vi "Enclose with Diagram Disable Structure Target.vi"(11 "Input":bool[](array[boolean])) -> (3 "Any?":bool)   [LabVIEW 2018, in "Tests.lvlib" / "Toolkit.lvlib" / "Unit.lvlib"]
uses:
  Unit.lvlib
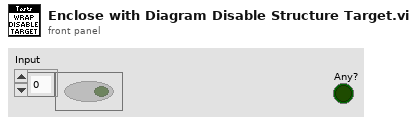
[diagram p1: front panel]
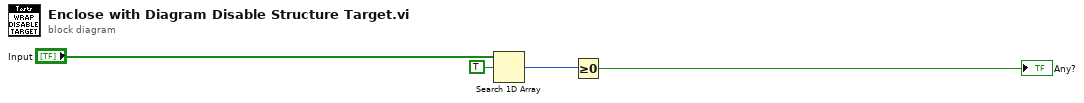
[diagram p0: block diagram]
diagram:
  n1 = Search 1D Array(1D array="Input", element=TRUE) -> (index of element=w1:i32)  [unwired: 1 in]
  n2 = Greater Or Equal To 0?(x=w1) -> (x >= 0?=→"Any?":bool)
